vi "auto_v2.vi"() -> ()   [LabVIEW 2012]
uses:
  SubVIs/State_Typ.ctl
  <vilib>/NXT/Hardware/Plugins/Tetrix DC Motor/TetrixDCMotorAddress.ctl
  SubVIs/auto_drive_TYP.ctl
  <vilib>/NXT/Dual Mode Library/Waits/Wait_Num(msec).vi
  <vilib>/NXT/NXTIO Xnodes/NXTIONodeSubVIs/TETRIX IO Check Battery.vi
  <vilib>/NXT/Dual Mode Library/Display/drawNumber.vi
  <vilib>/NXT/NXTIO Xnodes/NXTIONodeSubVIs/TETRIX IO Stop DC Motors.vi
  <vilib>/NXT/Dual Mode Library/Sound/Tone.vi
  <vilib>/NXT/Dual Mode Library/Waits/Wait_Num.vi
  <vilib>/NXT/Subs/LVHSConnector.ctl
  <vilib>/NXT/NXTIO Xnodes/AddressXNode/NXTIOAddress.xnode
  <vilib>/NXT/NXTIO Xnodes/NXTIOXNode/NXTIO.xnode
  Mecanum Drive.lvrbt
  <vilib>/NXT/LegoClasses/BrickReference/BrickReference.lvclass
panel:
  out "Enabled":bool
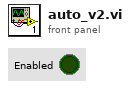
[diagram p1: front panel]
types:
  T1 = typedef "State_Typ.ctl" = enum16{"Stop", "Check for Position 3", "Check for Position 2", "Move to Pos 1", "Move to Pos 2", "Move to Pos 3"}
  T2 = typedef "TetrixDCMotorAddress.ctl" = i32
  T3 = typedef "LVHSConnector.ctl" = refnum<class "BrickReference.lvclass">
  T4 = cluster{"TetrixDCMotor":T2, "TetrixDCMotor 2":T2}
  T5 = typedef "auto_drive_TYP.ctl" = cluster{"Left X":i8, "Left Y":i8, "Right X":i8, "Power (100)":i8, "Wait (ms)":u32}
  T6 = cluster{"Direction (0-9)":i16, "Signal Strength (Array)":u8[]}
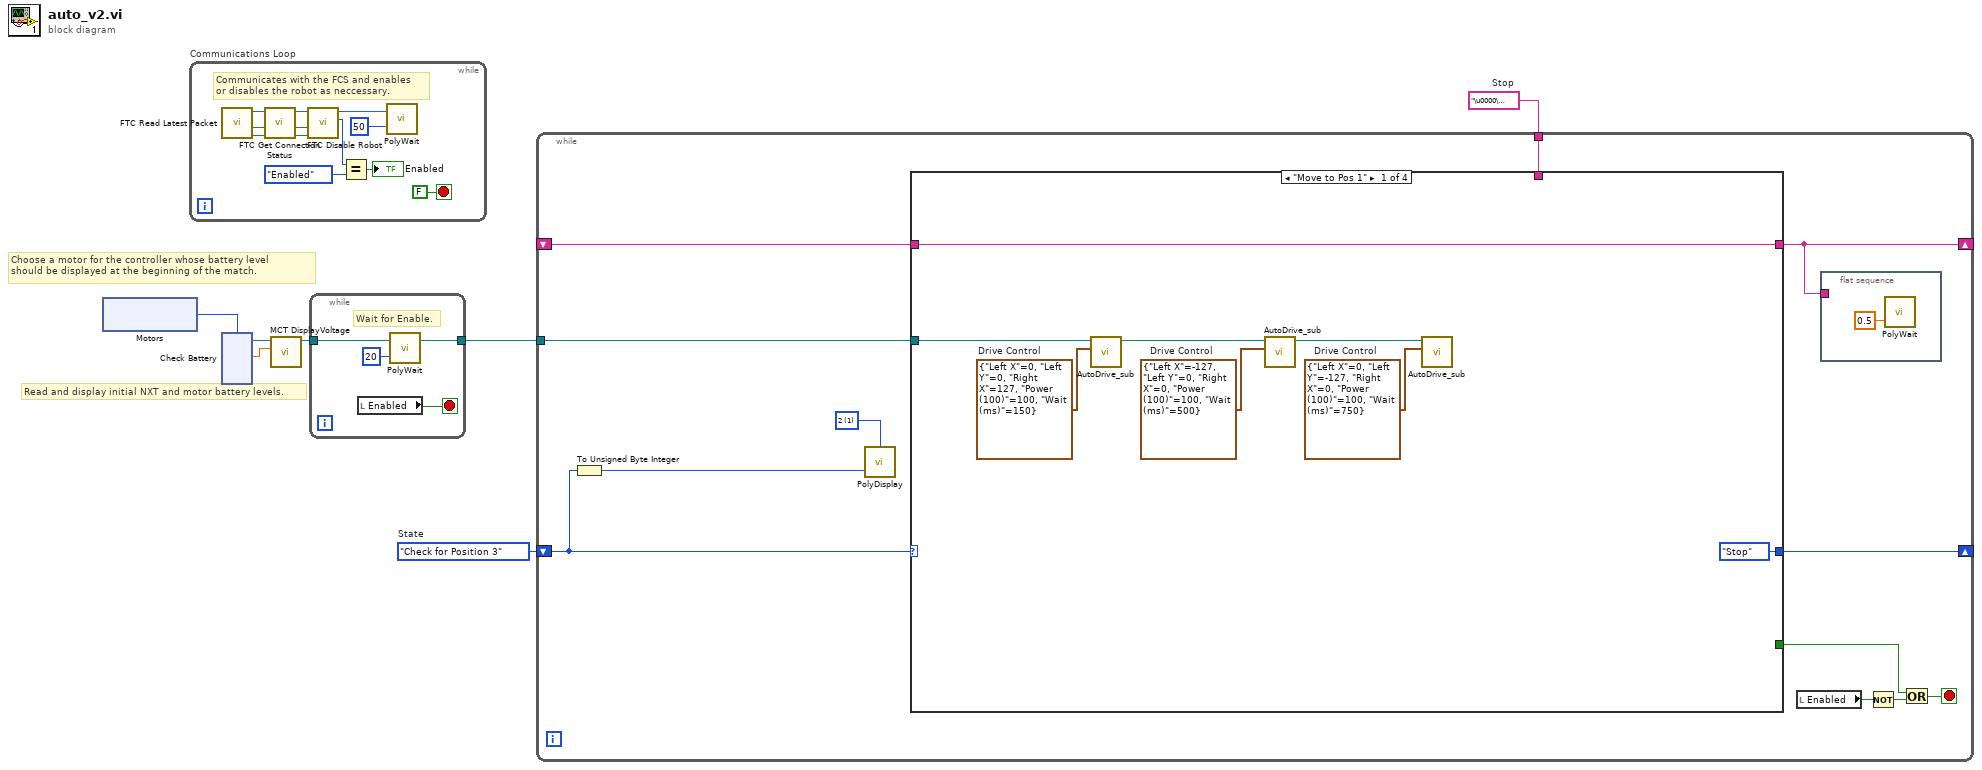
[diagram p0: block diagram]
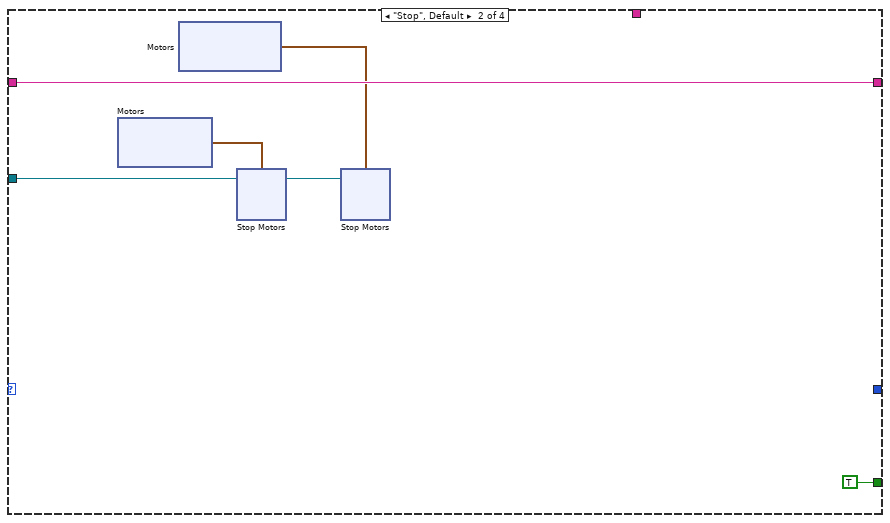
[diagram p2: hidden frame]
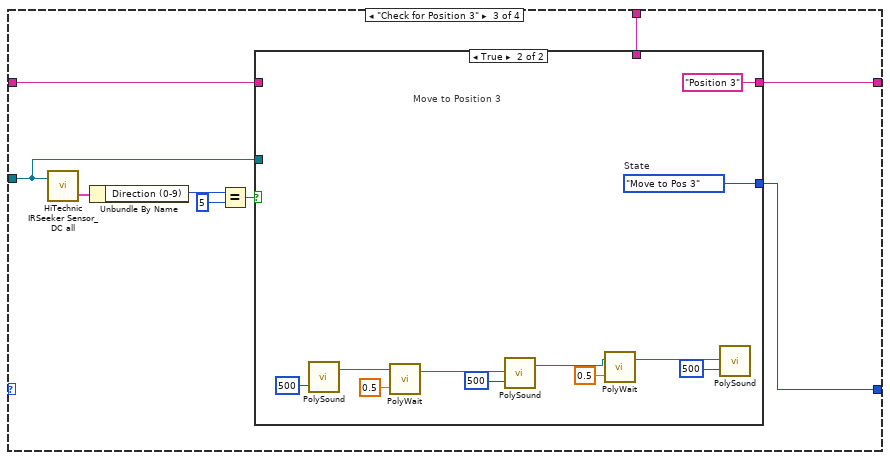
[diagram p3: hidden frame]
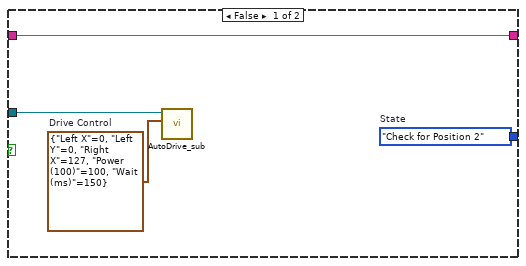
[diagram p4: hidden frame]
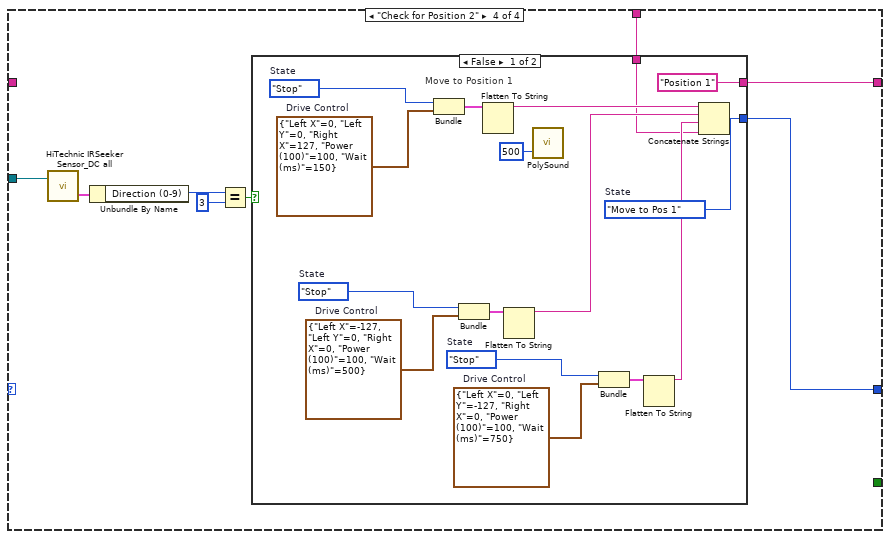
[diagram p5: hidden frame]
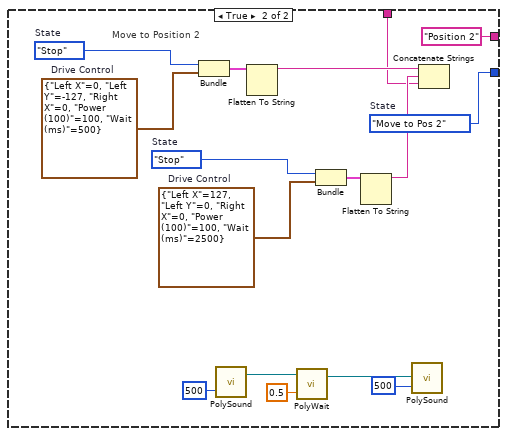
[diagram p6: hidden frame]
diagram:
  w6 = "\u0000\u0003\u0000\u0000d\u0000\u0000\u0000–"  # Stop
  w1 = State_Typ."Check for Position 3"  # State
  # "Read and display initial NXT and motor battery levels."
  # "Choose a motor for the controller whose battery level \nshould be displayed at the beginning of the match."
  n1 = xnode "Motors"() -> ("Motor"=w2:T2)
  n2 = while "Communications Loop" {
    stop <- FALSE stop-if-true
    # "Communicates with the FCS and enables \nor disables the robot as neccessary."
    n3 = call <vilib>:"FTC Read Latest Packet.vi"() -> ("Packet Received?"=w17:bool, "Stopped?"=w16:bool, "NXT"=w19:T3)  [unwired: 6 in, 3 out]
    n4 = call <vilib>:"FTC Get Connection Status.vi"("Packet Received?"=w17, "Stopped?"=w16, "NXT"=w19) -> ("Online?"=w8:bool, "Stopped?"=w9:bool, "NXT"=w18:T3)  [unwired: 5 in]
    n5 = call <vilib>:"FTC Disable Robot.vi"("Online?"=w8, "Stopped?"=w9, "NXT"=w18) -> ("Enabled?"=w12:enum16{"Disabled", "Enabled"}, "NXT"=w14:T3)  [unwired: 3 in]
    n6 = Equal?(x=w12, y=enum16{"Disabled", "Enabled"}."Enabled") -> (x = y?=→"Enabled":bool)
    n7 = call-poly <vilib>:"PolyWait.vi"("Time (100 msec)"=u32 50 ("Time (msec)"), "NXT/EV3"=w14) -> ()  [unwired: 2 in, 1 out]
  }
  n8 = xnode "Check Battery"("Motors"=w2) -> ("Voltage 1"=w3:sgl, "NXT/EV3"=w5:T3)  [unwired: 1 in]
  n9 = call <vilib>:"MCT DisplayVoltage.vi"("Motor Voltage"=w3, "NXT"=w5) -> ("NXT"=w4:T3)  [unwired: 9 in]
  n10 = while {
    tunnel: [w21] -> w7
    tunnel: w4 -> [w20]
    stop <- w22 stop-if-true
    # "Wait for Enable."
    n11 = local read "Enabled"() -> (w22:bool)
    n12 = call-poly <vilib>:"PolyWait.vi"("Time (100 msec)"=u32 20 ("Time (msec)"), "NXT/EV3"=w20) -> ("NXT/EV3"=w21:T3)  [unwired: 2 in]
  }
  n13 = while {
    tunnel: w7 -> [w35]
    shift-right: [w31] -> _
    shift-left: w1 -> [w25]
    shift-right: [w26] -> _
    shift-left: _ -> [w30]
    tunnel: w6 -> [w29]
    stop <- w34 stop-if-true
    w27 = i16 1 items=["1", "2", "3", "4", "5", "6", "7", "8", "9", "10", "11", "12"] ("Line")
    n14 = To Unsigned Byte Integer(number=w25) -> (unsigned 8bit integer=w24:u8)
    n15 = call-poly <vilib>:"PolyDisplay.vi"("number"=w24, "Line"=w27) -> ()  [unwired: 2 in, 1 out]
    n16 = case shown="\"Move to Pos 1\"" w25 {
      tunnel: w35 -> [w37 w50 w63 w91]
      tunnel: [_ TRUE _ _] -> w33
      tunnel: [State_Typ."Stop" ("State") _ w64 w87] -> w31
      tunnel: [w44 w48 w67 w89] -> w26
      tunnel: w30 -> [w44 w48 w66 _]
      tunnel: w29 -> [_ _ w65 w88]
      frame "Move to Pos 1" {
        w41 = T5 {"Left X"=-127, "Left Y"=0, "Right X"=0, "Power (100)"=100, "Wait (ms)"=500}  # Drive Control
        w38 = T5 {"Left X"=0, "Left Y"=-127, "Right X"=0, "Power (100)"=100, "Wait (ms)"=750}  # Drive Control
        w42 = T5 {"Left X"=0, "Left Y"=0, "Right X"=127, "Power (100)"=100, "Wait (ms)"=150}  # Drive Control
        n17 = call "AutoDrive_sub.vi"("Drive Control"=w42, "NXT/EV3"=w37) -> ("NXT/EV3 out"=w40:T3)  [unwired: 9 in]
        n18 = call "AutoDrive_sub.vi"("Drive Control"=w41, "NXT/EV3"=w40) -> ("NXT/EV3 out"=w39:T3)  [unwired: 9 in]
        n19 = call "AutoDrive_sub.vi"("Drive Control"=w38, "NXT/EV3"=w39) -> ()  [unwired: 9 in, 1 out]
      }
      frame "Stop", Default {
        n20 = xnode "Motors"() -> ("Motor"=w47:cluster{"TetrixDCMotor":T2, "TetrixDCMotor":T2})
        n21 = xnode "Motors"() -> ("Motor"=w46:cluster{"TetrixDCMotor":T2, "TetrixDCMotor":T2})
        n22 = xnode "Stop Motors"("Motors"=w47, "NXT/EV3"=w50) -> ("NXT/EV3"=w45:T3)
        n23 = xnode "Stop Motors"("Motors"=w46, "NXT/EV3"=w45) -> ()  [unwired: 1 out]
      }
      frame "Check for Position 3" {
        n24 = call <vilib>:"HiTechnic IRSeeker Sensor_DC all.vi"("NXT/EV3"=w63) -> ("All Info"=w71:T6)  [unwired: 2 in, 1 out]
        n25 = Unbundle By Name(w71) -> ("Direction (0-9)"=w69:i16)
        n26 = Equal?(x=w69, y=i16 5) -> (x = y?=w68:bool)
        n27 = case shown="True" w68 {
          tunnel: [w74 w76] -> w64
          tunnel: [w75 "Position 3"] -> w67
          tunnel: w66 -> [w75 _]
          tunnel: w65 -> [_ _]
          tunnel: w63 -> [w72 _]
          frame False {
            w73 = T5 {"Left X"=0, "Left Y"=0, "Right X"=127, "Power (100)"=100, "Wait (ms)"=150}  # Drive Control
            w74 = State_Typ."Check for Position 2"  # State
            n28 = call "AutoDrive_sub.vi"("Drive Control"=w73, "NXT/EV3"=w72) -> ()  [unwired: 9 in, 1 out]
          }
          frame True {
            w76 = State_Typ."Move to Pos 3"  # State
            # "Move to Position 3"
            n29 = call-poly <vilib>:"PolySound.vi"("Duration (500 ms)"=u16 500) -> ("NXT/EV3"=w82:T3)  [unwired: 3 in]
            n30 = call-poly <vilib>:"PolyWait.vi"("Time (1 sec)"=sgl 0.5, "NXT/EV3"=w82) -> ("NXT/EV3"=w81:T3)  [unwired: 2 in]
            n31 = call-poly <vilib>:"PolySound.vi"("Duration (500 ms)"=u16 500, "NXT/EV3"=w81) -> ("NXT/EV3"=w78:T3)  [unwired: 2 in]
            n32 = call-poly <vilib>:"PolyWait.vi"("Time (1 sec)"=sgl 0.5, "NXT/EV3"=w78) -> ("NXT/EV3"=w77:T3)  [unwired: 2 in]
            n33 = call-poly <vilib>:"PolySound.vi"("Duration (500 ms)"=u16 500, "NXT/EV3"=w77) -> ()  [unwired: 2 in, 1 out]
          }
        }
      }
      frame "Check for Position 2" {
        n34 = call <vilib>:"HiTechnic IRSeeker Sensor_DC all.vi"("NXT/EV3"=w91) -> ("All Info"=w94:T6)  [unwired: 2 in, 1 out]
        n35 = Unbundle By Name(w94) -> ("Direction (0-9)"=w92:i16)
        n36 = Equal?(x=w92, y=i16 3) -> (x = y?=w90:bool)
        n37 = case shown="False" w90 {
          tunnel: [w95 w111] -> w87
          tunnel: ["Position 1" "Position 2"] -> w89
          tunnel: w88 -> [w96 w112]
          frame False {
            w95 = State_Typ."Move to Pos 1"  # State
            w103 = T5 {"Left X"=-127, "Left Y"=0, "Right X"=0, "Power (100)"=100, "Wait (ms)"=500}  # Drive Control
            w104 = State_Typ."Stop"  # State
            w106 = T5 {"Left X"=0, "Left Y"=-127, "Right X"=0, "Power (100)"=100, "Wait (ms)"=750}  # Drive Control
            w107 = State_Typ."Stop"  # State
            w109 = T5 {"Left X"=0, "Left Y"=0, "Right X"=127, "Power (100)"=100, "Wait (ms)"=150}  # Drive Control
            w110 = State_Typ."Stop"  # State
            # "Move to Position 1"
            n38 = Bundle("State"=w110, "Drive Control"=w109) -> (w108:cluster{"State":T1, "Drive Control":T5})  [unwired: 1 in]
            n39 = Bundle("State"=w104, "Drive Control"=w103) -> (w102:cluster{"State":T1, "Drive Control":T5})  [unwired: 1 in]
            n40 = Flatten To String(anything=w108) -> (data string=w98:string)  [unwired: 3 in, 2 out]
            n41 = Flatten To String(anything=w102) -> (data string=w101:string)  [unwired: 3 in, 2 out]
            n42 = call-poly <vilib>:"PolySound.vi"("Duration (500 ms)"=u16 500) -> ()  [unwired: 3 in, 1 out]
            n43 = Bundle("State"=w107, "Drive Control"=w106) -> (w105:cluster{"State":T1, "Drive Control":T5})  [unwired: 1 in]
            n44 = Flatten To String(anything=w105) -> (data string=w100:string)  [unwired: 3 in, 2 out]
            n45 = Concatenate Strings(w98, w101, w100, w96) -> ()  [unwired: 1 out]
          }
          frame True {
            w111 = State_Typ."Move to Pos 2"  # State
            w122 = T5 {"Left X"=127, "Left Y"=0, "Right X"=0, "Power (100)"=100, "Wait (ms)"=2500}  # Drive Control
            w121 = State_Typ."Stop"  # State
            w119 = T5 {"Left X"=0, "Left Y"=-127, "Right X"=0, "Power (100)"=100, "Wait (ms)"=500}  # Drive Control
            w120 = State_Typ."Stop"  # State
            # "Move to Position 2"
            n46 = Bundle("State"=w120, "Drive Control"=w119) -> (w123:cluster{"State":T1, "Drive Control":T5})  [unwired: 1 in]
            n47 = call-poly <vilib>:"PolySound.vi"("Duration (500 ms)"=u16 500) -> ("NXT/EV3"=w114:T3)  [unwired: 3 in]
            n48 = Flatten To String(anything=w123) -> (data string=w126:string)  [unwired: 3 in, 2 out]
            n49 = call-poly <vilib>:"PolyWait.vi"("Time (1 sec)"=sgl 0.5, "NXT/EV3"=w114) -> ("NXT/EV3"=w113:T3)  [unwired: 2 in]
            n50 = Bundle("State"=w121, "Drive Control"=w122) -> (w124:cluster{"State":T1, "Drive Control":T5})  [unwired: 1 in]
            n51 = Flatten To String(anything=w124) -> (data string=w125:string)  [unwired: 3 in, 2 out]
            n52 = call-poly <vilib>:"PolySound.vi"("Duration (500 ms)"=u16 500, "NXT/EV3"=w113) -> ()  [unwired: 2 in, 1 out]
            n53 = Concatenate Strings(w126, w125, w112) -> ()  [unwired: 1 out]
          }
        }
      }
    }
    n54 = local read "Enabled"() -> (w32:bool)
    n55 = flat-sequence {
      tunnel: w26 -> [_]
      frame #0 {
        n56 = call-poly <vilib>:"PolyWait.vi"("Time (1 sec)"=sgl 0.5) -> ()  [unwired: 3 in, 1 out]
      }
    }
    n57 = Not(x=w32) -> (.not. x?=w28:bool)
    n58 = Or(x=w33, y=w28) -> (x .or. y?=w34:bool)
  }
